vi "Validate channels.vi"(7 "application reference (local)":refnum<vi>, 8 "error in (no error)":errorcluster, 11 "data ctl":string[](array[string])) -> (0 "error out":errorcluster)   [LabVIEW 2013, in "control module data interface generator.lvlib"]
uses:
  control module data interface generator.lvlib
  DefaultsGlobal.vi
  <vilib>/regexp/Match Regular Expression.xnode
  <vilib>/Utility/VariantDataType/VariantType.lvlib
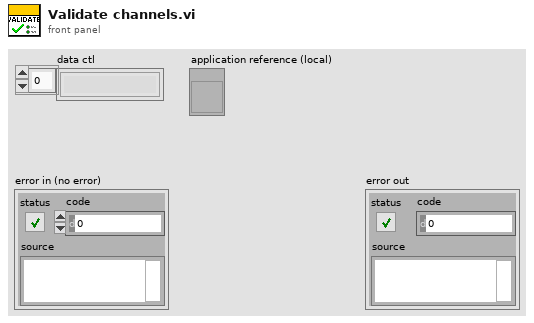
[diagram p1: front panel]
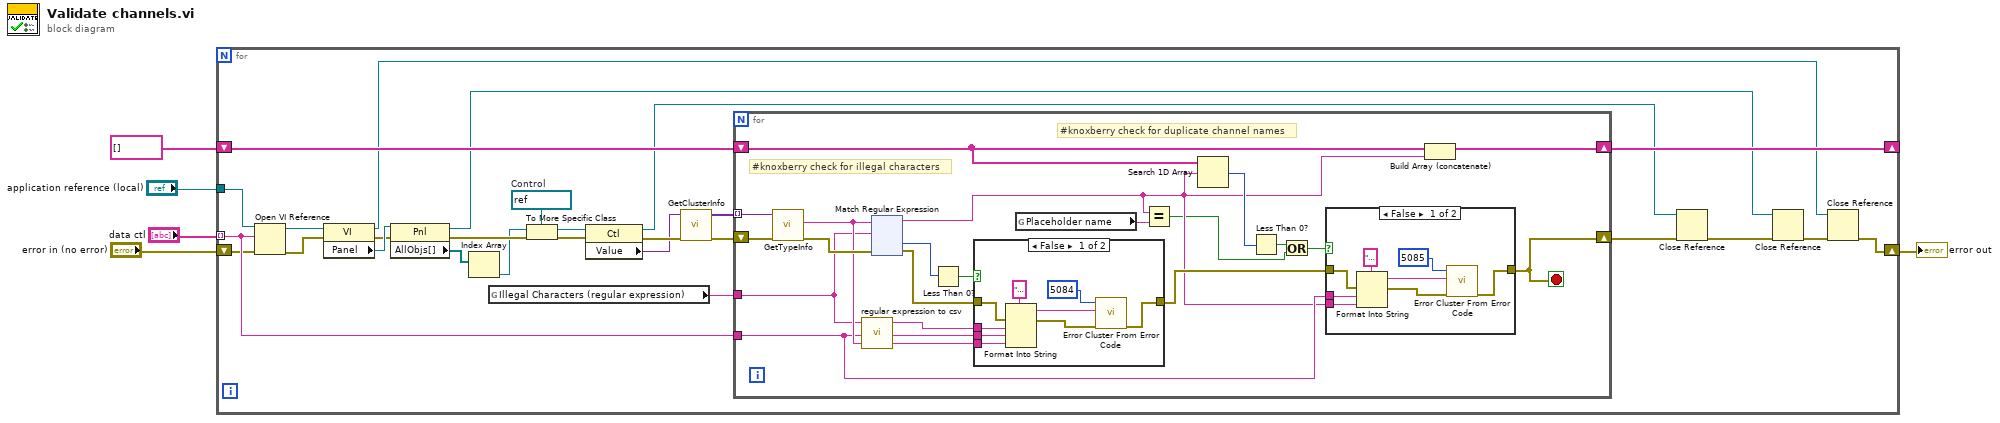
[diagram p0: block diagram]
diagram:
  n1 = for {
    tunnel: "data ctl" -> [w16] mode=indexing
    tunnel: "application reference (local)" -> [w32]
    shift-right: [w11] -> w1
    shift-left: "error in (no error)" -> [w15]
    shift-right: [w14] -> _
    shift-left: string[] [] -> [w13]
    w24 = refnum<vi> refnum  # Control
    n2 = Open VI Reference(application reference (local)=w32, vi path=w16, error in (no error)=w15) -> (vi reference=w31:refnum<vi>, error out=w30:errorcluster)  [unwired: 3 in]
    n3 = property class="VI"(reference=w31, error in=w30) -> (reference out=w10:refnum<vi>, error out=w28:errorcluster, "Panel"=w29:refnum<vi>)
    n4 = property class="Pnl"(reference=w29, error in=w28) -> (reference out=w9:refnum<vi>, error out=w26:errorcluster, "AllObjs[]"=w27:refnum<vi>[])
    n5 = Index Array(array=w27) -> (element=w25:refnum<vi>)  [unwired: 1 in]
    n6 = global read "DefaultsGlobal.vi" "Illegal Characters (regular expression)"() -> (w17:string)
    n7 = To More Specific Class(target class=w24, reference=w25, error in=w26) -> (specific class reference=w23:refnum<vi>, error out=w22:errorcluster)
    n8 = property class="Ctl"(reference=w23, error in=w22) -> (reference out=w6:refnum<vi>, error out=w21:errorcluster, "Value"=w20:variant)
    n9 = call <vilib>:"GetClusterInfo.vi"("error in (no error)"=w21, "Variant"=w20) -> ("error out"=w18:errorcluster, "Cluster Elements"=w19:variant[])  [unwired: 8 in]
    n10 = for {
      tunnel: w19 -> [w52] mode=indexing
      shift-right: [w38] -> w8
      shift-left: w18 -> [w51]
      shift-right: [w46] -> w14
      shift-left: w13 -> [w47]
      tunnel: w17 -> [w42]
      tunnel: w16 -> [w40]
      stop <- w38 stop-if-true
      # "#knoxberry check for duplicate channel names"
      # "#knoxberry check for illegal characters"
      n11 = call <vilib>:"GetTypeInfo.vi"("error in (no error)"=w51, "Variant"=w52) -> ("error out"=w50:errorcluster, "Name"=w43:string)  [unwired: 5 in, 3 out]
      n12 = call "regular expression to csv.vi"("regular expression"=w42) -> ("csv"=w41:string)  [unwired: 10 in]
      n13 = xnode "Match Regular Expression"("input string"=w43, "regular expression"=w42, "error in"=w50) -> ("before match"=w36:string, "offset past match"=w49:i32, "error out"=w44:errorcluster)  [unwired: 3 in, 2 out]
      n14 = Less Than 0?(x=w49) -> (x < 0?=w45:bool)
      n15 = case shown="False" w45 {
        tunnel: w44 -> [w67 w71]
        tunnel: w40 -> [w68 _]
        tunnel: w43 -> [w66 _]
        tunnel: w41 -> [w65 _]
        tunnel: [w62 w71] -> w39
        frame False {
          n16 = Format Into String(format string="An illegal character was discovered in a channel name during validation. Illegal characters include: %s\n\nControl: %s\nName: %s" ("Name"), error in=w67, w65, w68, w66) -> (resulting string=w64:string, error out=w63:errorcluster)  [unwired: 1 in]
          n17 = call <vilib>:"Error Cluster From Error Code.vi"("error in (no error)"=w63, "error message (\"\")"=w64, "error code (0)"=5084) -> ("error out"=w62:errorcluster)  [unwired: 6 in]
        }
        frame True {
        }
      }
      n18 = global read "DefaultsGlobal.vi" "Placeholder name"() -> (w37:string)
      n19 = Equal?(x=w36, y=w37) -> (x = y?=w34:bool)
      n20 = Search 1D Array(1D array=w47, element=w36) -> (index of element=w48:i32)  [unwired: 1 in]
      n21 = Less Than 0?(x=w48) -> (x < 0?=w35:bool)
      n22 = Or(x=w35, y=w34) -> (x .or. y?=w33:bool)
      n23 = case shown="False" w33 {
        tunnel: w39 -> [w57 w61]
        tunnel: w36 -> [w58 _]
        tunnel: w40 -> [w56 _]
        tunnel: [w53 w61] -> w38
        frame False {
          n24 = Format Into String(format string="A duplicate channel name was discovered during validation. All channels in a module must contain unique names.\n\nControl: %s\nName: %s" ("Name"), error in=w57, w56, w58) -> (resulting string=w55:string, error out=w54:errorcluster)  [unwired: 1 in]
          n25 = call <vilib>:"Error Cluster From Error Code.vi"("error in (no error)"=w54, "error message (\"\")"=w55, "error code (0)"=5085) -> ("error out"=w53:errorcluster)  [unwired: 6 in]
        }
        frame True {
        }
      }
      n26 = Build Array (concatenate)(w47, w36) -> (w46:string[])
    }
    n27 = Close Reference(reference=w6, error in (no error)=w8) -> (error out=w7:errorcluster)
    n28 = Close Reference(reference=w9, error in (no error)=w7) -> (error out=w12:errorcluster)
    n29 = Close Reference(reference=w10, error in (no error)=w12) -> (error out=w11:errorcluster)
  }
  "error out" <- w1
